vi "Main.vi"(11 "Module Admin":refnum<class "Delacor_lib_QMH_Module Admin.lvclass">) -> ()   [LabVIEW 2020, in "UI.lvlib"]
doc: "This template is based off of the Queued Message Handler design pattern and the Queued Message Handler project template that ships with LabVIEW.\n\nThe main difference is that the queue is private to this module and communication between modules is performed via Broadcast and Request events.\n\nRequest events are wrapped in public API methods and are handled in the Event Handling Loop (EHL) of this VI. Any module can register for Broadcast events sent by this module. The EHL generates messages based on user interface actions.\n\nThe Message Handling Loop (MHL) processes messages generated by the EHL, or by other messages. The messages are string values, so new messages can be added easily to the Message Cases case structure in the MHL. Each message cluster can also provide an optional value for Message Data, which is a variant that can be converted to whatever message-specific data is required.\n_____\nBased on Delacor QMH Project Template 5.0.0.82."
uses:
  UI.lvlib
  <vilib>/Delacor/Delacor QMH/Libraries/Module Admin_class/Delacor_lib_QMH_Module Admin.lvclass
  Module Data--cluster.ctl
  Stop Argument--cluster.ctl
  <vilib>/Delacor/Delacor QMH/Libraries/Message Queue_class/Delacor_lib_QMH_Message Queue.lvclass/Delacor_lib_QMH_Message Queue.ctl
  <vilib>/Delacor/Delacor QMH/Libraries/Module Admin_class/Delacor_lib_QMH_Module Admin.lvclass/Delacor_lib_QMH_Module Admin.ctl
  <vilib>/Delacor/Delacor QMH/Libraries/Message Queue_class/Delacor_lib_QMH_Enqueue Message (Single).vi
  <vilib>/Delacor/Delacor QMH/Libraries/Module Admin_class/Delacor_lib_QMH_Get External Launch.vi
  <vilib>/Utility/error.llb/Error Cluster From Error Code.vi
  <vilib>/ErrorRing/Error Ring.xnode
  <vilib>/Delacor/Delacor QMH/Libraries/Message Queue_class/Delacor_lib_QMH_Message Queue.lvclass
  Productos/Productos.lvlib
  Monedas/Monedas.lvlib
  Mensajes/Mensajes.lvlib
panel:
  out "error out":errorcluster
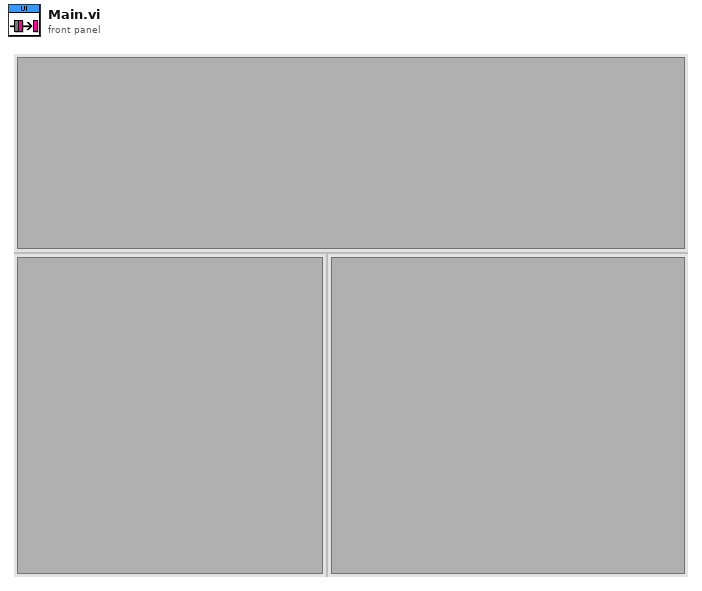
[diagram p1: front panel]
types:
  T1 = typedef "UI.lvlib/Request Events--cluster.ctl" = cluster{"Stop Module":refnum<user-event>, "Show Panel":refnum<user-event>, "Hide Panel":refnum<user-event>, "Get Module Execution Status":refnum<user-event>, "Show Diagram":refnum<user-event>}
  T2 = typedef "Mensajes.lvlib/Broadcast Events--cluster.ctl" = cluster{"Module Did Init":refnum<user-event>, "Status Updated":refnum<user-event>, "Error Reported":refnum<user-event>, "Module Did Stop":refnum<user-event>, "Update Module Execution Status":refnum<user-event>}
  T3 = typedef "Monedas.lvlib/Broadcast Events--cluster.ctl" = cluster{"Module Did Init":refnum<user-event>, "Status Updated":refnum<user-event>, "Error Reported":refnum<user-event>, "Module Did Stop":refnum<user-event>, "Update Module Execution Status":refnum<user-event>}
  T4 = typedef "Productos.lvlib/Broadcast Events--cluster.ctl" = cluster{"Module Did Init":refnum<user-event>, "Status Updated":refnum<user-event>, "Error Reported":refnum<user-event>, "Module Did Stop":refnum<user-event>, "Update Module Execution Status":refnum<user-event>}
  T5 = typedef "UI.lvlib/Module Data--cluster.ctl" = cluster{"Status":string}
  T6 = enum32{"invalid lock state", "Not Locked", "Locked (No Password)", "Password-protected"}
  T7 = typedef "UI.lvlib/Stop Argument--cluster.ctl" = cluster{"Origin":string, "Exit via Stop Module Req?":bool, "Wait for Module to stop?":bool}
  T8 = enum32{"Invalid", "Standard", "Closed", "Hidden", "Minimized", "Maximized"}
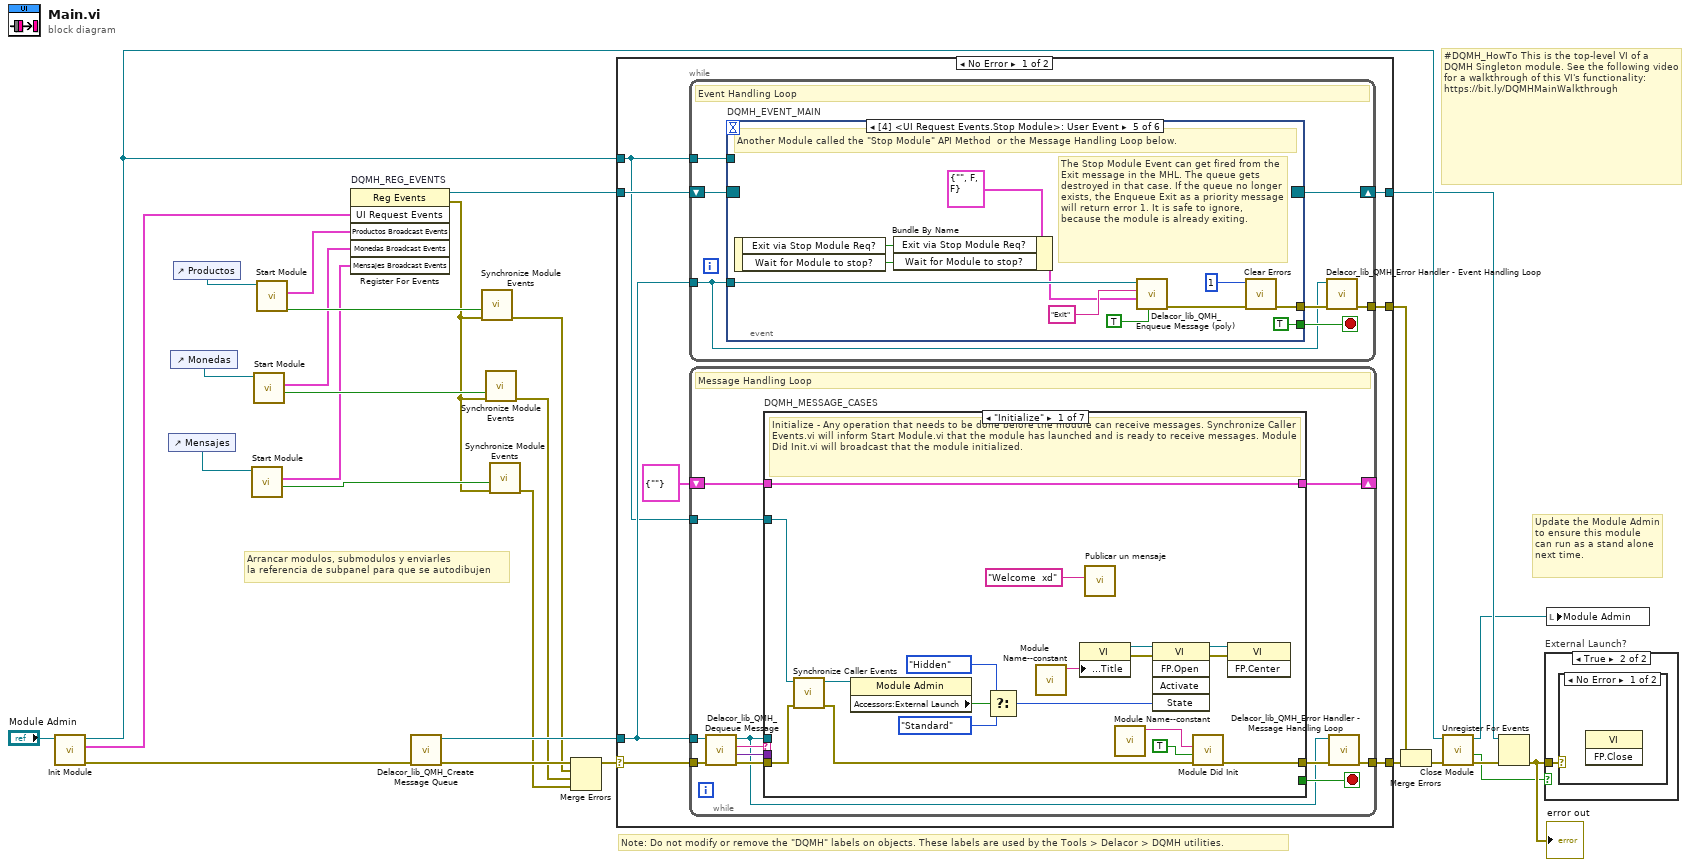
[diagram p0: block diagram]
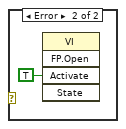
[diagram p3: hidden frame]
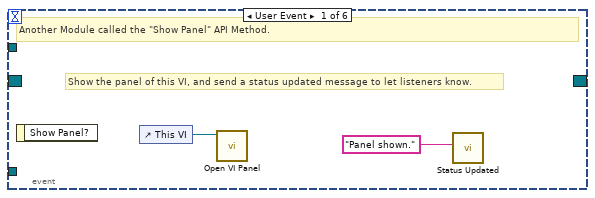
[diagram p4: hidden frame]
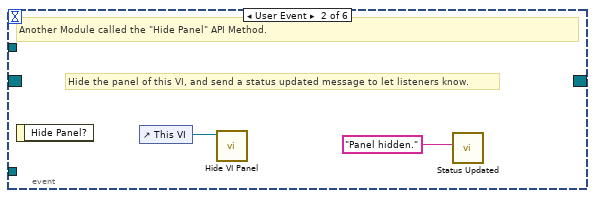
[diagram p5: hidden frame]
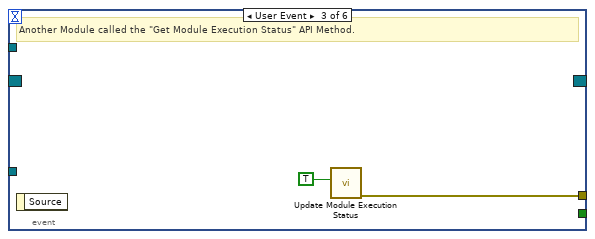
[diagram p6: hidden frame]
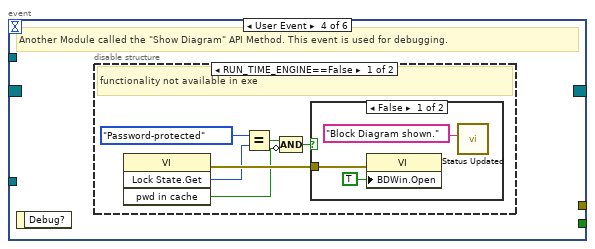
[diagram p7: hidden frame]
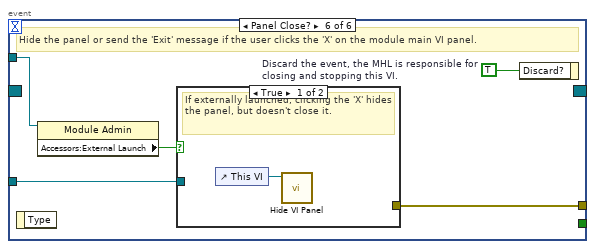
[diagram p10: hidden frame]
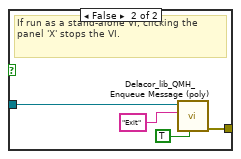
[diagram p11: hidden frame]
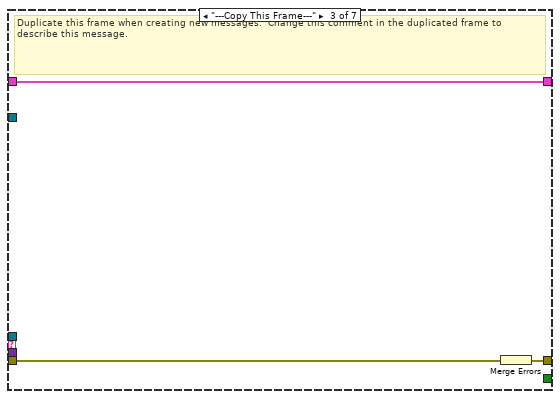
[diagram p13: hidden frame]
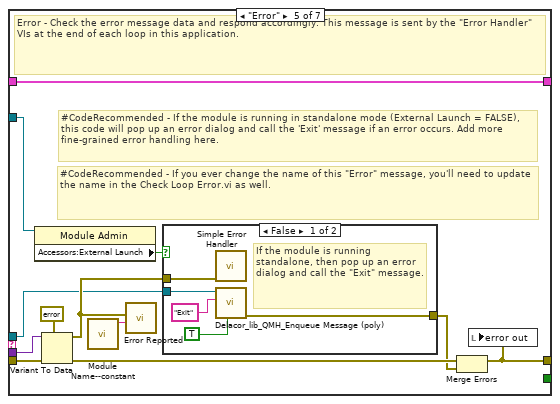
[diagram p15: hidden frame]
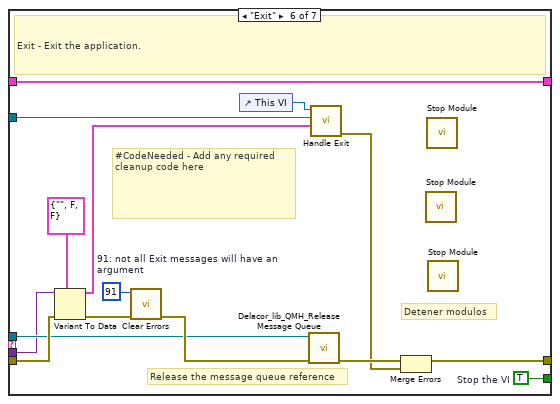
[diagram p17: hidden frame]
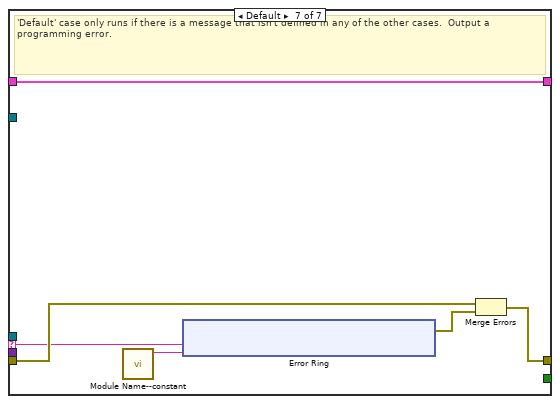
[diagram p18: hidden frame]
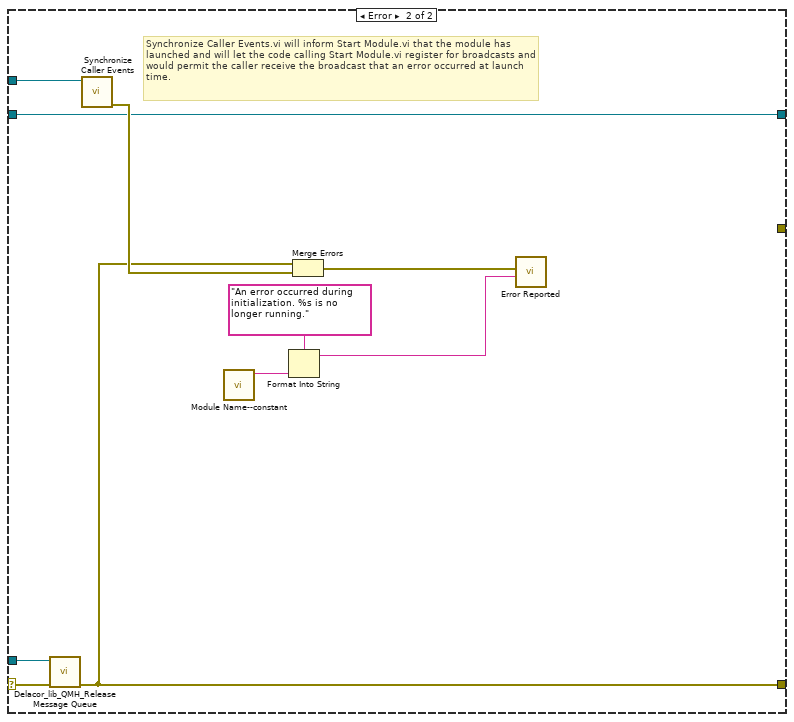
[diagram p19: hidden frame]
diagram:
  # "Arrancar modulos, submodulos y enviarles\nla referencia de subpanel para que se autodibujen"
  # "#DQMH_HowTo This is the top-level VI of a DQMH Singleton module. See the following video for a walkthrough of this VI's functionality: https://bit.ly/DQMHMainWalkthrough"
  # "Note: Do not modify or remove the \"DQMH\" labels on objects. These labels are used by the Tools > Delacor > DQMH utilities."
  # "Update the Module Admin to ensure this module can run as a stand alone next time."
  n1 = call "Init Module.vi"("Singleton Module Admin in"="Module Admin") -> ("error out"=w28:errorcluster, "UI Request Events"=w18:T1, "Singleton Module Admin out"=w21:refnum<class "Delacor_lib_QMH_Module Admin.lvclass">)  [unwired: 8 in]
  n2 = control-ref of="Mensajes"() -> (w7:refnum<vi>)
  n3 = control-ref of="Monedas"() -> (w10:refnum<vi>)
  n4 = control-ref of="Productos"() -> (w13:refnum<vi>)
  n5 = call "Start Module.vi"("Mensajes"=w7) -> ("Wait for Event Sync?"=w5:bool, "Mensajes Broadcast Events"=w6:T2)  [unwired: 7 in, 2 out]
  n6 = call "Start Module.vi"("Monedas"=w10) -> ("Wait for Event Sync?"=w8:bool, "Monedas Broadcast Events"=w9:T3)  [unwired: 7 in, 2 out]
  n7 = call "Start Module.vi"("Productos"=w13) -> ("Wait for Event Sync?"=w11:bool, "Productos Broadcast Events"=w12:T4)  [unwired: 7 in, 2 out]
  n8 = register-events "DQMH_REG_EVENTS"(w18, w12, w9, w6) -> (reference out=w19:refnum<event-registration>, error out=w4:errorcluster)  [unwired: 2 in]
  n9 = call <vilib>:"Delacor_lib_QMH_Create Message Queue.vi"("error in (no error)"=w28) -> ("error out"=w23:errorcluster, "Message Queue"=w17:refnum<class "Delacor_lib_QMH_Message Queue.lvclass">)  [unwired: 9 in]
  n10 = call "Synchronize Module Events.vi"("error in (no error)"=w4, "Wait for Event Sync?"=w11) -> ("error out"=w3:errorcluster)  [unwired: 9 in]
  n11 = call "Synchronize Module Events.vi"("error in (no error)"=w4, "Wait for Event Sync?"=w8) -> ("error out"=w2:errorcluster)  [unwired: 9 in]
  n12 = call "Synchronize Module Events.vi"("error in (no error)"=w4, "Wait for Event Sync?"=w5) -> ("error out"=w1:errorcluster)  [unwired: 9 in]
  n13 = Merge Errors(w23, w3, w2, w1) -> (w22:errorcluster)
  n14 = case shown="No Error" w22 {
    selector: w22 -> [w35 w166]
    tunnel: [w37 w165] -> w29
    tunnel: [w34 w171] -> w20
    tunnel: w19 -> [w32 w171]
    tunnel: w17 -> [w31 w164]
    tunnel: [w36 _] -> w26
    tunnel: w21 -> [w30 w167]
    frame No Error {
      n15 = while {
        tunnel: w31 -> [w38]
        shift-right: [w41] -> w34
        shift-left: w32 -> [w42]
        tunnel: [w43] -> w36
        tunnel: w30 -> [w39]
        stop <- w40 stop-if-true
        # "Event Handling Loop"
        n16 = event "DQMH_EVENT_MAIN" shown="[4] <UI Request Events.Stop Module>: User Event" {
          selector: w42 -> [_ _ _ _ _ _]
          dyn-events: [_ _ _ _ _ _] -> w41
          timeout: _ -> [_ _ _ _ _ _]
          tunnel: [_ _ _ _ TRUE ("Discard?") _] -> w40
          tunnel: w38 -> [_ _ _ _ w66 w73]
          tunnel: [_ _ w50 _ w69 w75] -> w44
          tunnel: w39 -> [_ _ _ _ _ w72]
          event User Event {
            # "Show the panel of this VI, and send a status updated message to let listeners know."
            # "Another Module called the \"Show Panel\" API Method."
            n17 = event-data() -> ()  [unwired: 1 in, 1 out]
            n18 = control-ref of="This VI"() -> (w46:refnum<vi>)
            n19 = call "Open VI Panel.vi"("VI"=w46) -> ()  [unwired: 10 in, 1 out]
            n20 = call "Status Updated.vi"("Status"="Panel shown." ("format string")) -> ()  [unwired: 10 in, 1 out]
          }
          event User Event {
            # "Hide the panel of this VI, and send a status updated message to let listeners know."
            # "Another Module called the \"Hide Panel\" API Method."
            n21 = event-data() -> ()  [unwired: 1 in, 1 out]
            n22 = control-ref of="This VI"() -> (w48:refnum<vi>)
            n23 = call "Hide VI Panel.vi"("VI"=w48) -> ()  [unwired: 10 in, 1 out]
            n24 = call "Status Updated.vi"("Status"="Panel hidden." ("format string")) -> ()  [unwired: 10 in, 1 out]
          }
          event User Event {
            # "Another Module called the \"Get Module Execution Status\" API Method."
            n25 = event-data() -> ()  [unwired: 1 in, 1 out]
            n26 = call "Update Module Execution Status.vi"("Running?"=TRUE) -> ("error out"=w50:errorcluster)  [unwired: 10 in]
          }
          event User Event {
            # "Another Module called the \"Show Diagram\" API Method. This event is used for debugging."
            n27 = event-data() -> ()  [unwired: 1 in, 1 out]
            n28 = disable-structure shown="RUN_TIME_ENGINE==False" {
              frame condition #0 (active) {
                # "functionality not available in exe"
                n29 = invoke class="VI" method="Lock State.Get"() -> (error out=w56:errorcluster, "Get Lock State"=w55:T6, "pwd in cache"=w52:bool)  [unwired: 4 in, 1 out]
                n30 = Equal?(x=T6."Password-protected", y=w55) -> (x = y?=w53:bool)
                n31 = Compound Arithmetic op=AND(w53, invert w52) -> (w51:bool)
                n32 = case shown="False" w51 {
                  tunnel: w56 -> [w59 _]
                  frame False {
                    n33 = property class="VI"(error in=w59, "BDWin.Open"=TRUE ("Block Diagram Window:Open")) -> ()  [unwired: 1 in, 2 out]
                    n34 = call "Status Updated.vi"("Status"="Block Diagram shown." ("format string")) -> ()  [unwired: 10 in, 1 out]
                  }
                  frame True {
                    # "Password-protected VI, and the password is not in the cache. Do not show the diagram."
                  }
                }
              }
              frame condition #1 {
              }
            }
          }
          event User Event {
            # "The Stop Module Event can get fired from the Exit message in the MHL. The queue gets destroyed in that case. If the queue no longer exists, the Enqueue Exit as a priority message will return error 1. It is safe to ignore, because the module is already exiting."
            # "Another Module called the \"Stop Module\" API Method  or the Message Handling Loop below."
            n35 = event-data() -> ("Exit via Stop Module Req?"=w62:bool, "Wait for Module to stop?"=w61:bool)  [unwired: 1 in]
            n36 = Bundle By Name(cluster=T7 {"Origin"="", "Exit via Stop Module Req?"=FALSE, "Wait for Module to stop?"=FALSE} ("Stop Argument"), "Exit via Stop Module Req?"=w62, "Wait for Module to stop?"=w61) -> (w60:T7)
            n37 = call-poly <vilib>:"Delacor_lib_QMH_Enqueue Message (poly).vi"("Priority Message? (F)"=TRUE, "Message Data"=w60, "Message"="Exit", "Message Queue in"=w66) -> ("error out"=w70:errorcluster)  [unwired: 6 in, 1 out]
            n38 = call <vilib>:"Clear Errors.vi"("error in (no error)"=w70, "specific error code to clear (0: all)"=1) -> ("error out"=w69:errorcluster)  [unwired: 4 in, 1 out]
          }
          event Panel Close? {
            w74 = TRUE  # Discard the event, the MHL is responsible for closing and stopping this VI.
            # "Hide the panel or send the 'Exit' message if the user clicks the 'X' on the module main VI panel."
            n39 = event-data() -> ()  [unwired: 1 in, 1 out]
            n40 = property class="Module Admin"(reference=w72) -> ("Accessors:External Launch"=w71:bool)  [unwired: 1 in, 2 out]
            n41 = case shown="True" w71 {
              tunnel: w73 -> [_ w79]
              tunnel: [_ w80] -> w75
              frame True {
                # "If externally launched, clicking the 'X' hides the panel, but doesn't close it."
                n42 = control-ref of="This VI"() -> (w76:refnum<vi>)
                n43 = call "Hide VI Panel.vi"("VI"=w76) -> ()  [unwired: 10 in, 1 out]
              }
              frame False {
                # "If run as a stand-alone VI, clicking the panel 'X' stops the VI."
                n44 = call-poly <vilib>:"Delacor_lib_QMH_Enqueue Message (poly).vi"("Priority Message? (F)"=TRUE, "Message"="Exit", "Message Queue in"=w79) -> ("error out"=w80:errorcluster)  [unwired: 7 in, 1 out]
              }
            }
            n45 = event-data("Discard?"=w74) -> ()  [unwired: 1 in, 1 out]
          }
        }
        n46 = call-dynamic "Delacor_lib_QMH_Error Handler - Event Handling Loop.vi"("error in (no error)"=w44, "Message Queue in"=w38) -> ("dup error in"=w43:errorcluster)  [unwired: 8 in, 1 out]
      }
      n47 = while {
        tunnel: w31 -> [w83]
        shift-right: [w87] -> _
        shift-left: T5 {"Status"=""} ("Data Cluster") -> [w88]
        tunnel: w35 -> [w91]
        tunnel: [w89] -> w37
        tunnel: w30 -> [w81]
        stop <- w86 stop-if-true
        # "Message Handling Loop"
        n48 = call-dynamic "Delacor_lib_QMH_Dequeue Message.vi"("error in (no error)"=w91, "Message Queue in"=w83) -> ("error out"=w90:errorcluster, "Message Data"=w84:variant, "Message"=w85:string, "Message Queue out"=w82:refnum<class "Delacor_lib_QMH_Message Queue.lvclass">)  [unwired: 6 in]
        n49 = case "DQMH_MESSAGE_CASES" shown="\"Initialize\"" w85 {
          selector: w85 -> [_ _ _ _ _ _ w151]
          tunnel: w82 -> [_ _ _ _ w121 w143 _]
          tunnel: w90 -> [w108 w112 w115 w117 w128 w149 w153]
          tunnel: [w106 w112 w114 w117 w124 w146 w154] -> w92
          tunnel: w88 -> [w97 w111 w113 w116 w123 w142 w152]
          tunnel: [w97 w111 w113 w116 w123 w142 w152] -> w87
          tunnel: [_ _ _ _ _ w141 _] -> w86
          tunnel: w84 -> [_ _ _ _ w122 w140 _]
          tunnel: w81 -> [w98 _ _ _ w120 w135 _]
          frame "Initialize" {
            # "Initialize - Any operation that needs to be done before the module can receive messages. Synchronize Caller Events.vi will inform Start Module.vi that the module has launched and is ready to receive messages. Module Did Init.vi will broadcast that the module initialized."
            n50 = call "Synchronize Caller Events.vi"("error in (no error)"=w108, "Singleton Module Admin in"=w98) -> ("error out"=w107:errorcluster, "Singleton Module Admin out"=w94:refnum<class "Delacor_lib_QMH_Module Admin.lvclass">)  [unwired: 8 in]
            n51 = property class="Module Admin"(reference=w94) -> ("Accessors:External Launch"=w102:bool)  [unwired: 1 in, 2 out]
            n52 = Select(t=T8."Hidden" ("State"), s=w102, f=T8."Standard" ("State")) -> (s? t:f=w99:T8)
            n53 = call "Module Name--constant.vi"() -> ("Module Name"=w105:string)  [unwired: 11 in]
            n54 = property class="VI"("Front Panel.Title"=w105) -> (reference out=w104:refnum<vi>, error out=w110:errorcluster)  [unwired: 2 in]
            n55 = call "Publicar un mensaje.vi"("Mensaje"="Welcome  xd") -> ()  [unwired: 10 in, 1 out]
            n56 = call "Module Name--constant.vi"() -> ("Module Name"=w95:string)  [unwired: 11 in]
            n57 = invoke class="VI" method="FP.Open"(reference=w104, error in=w110, "State"=w99) -> (reference out=w103:refnum<vi>, error out=w109:errorcluster)  [unwired: 2 in, 3 out]
            n58 = call "Module Did Init.vi"("error in (no error)"=w107, "Initialized?"=TRUE, "Origin"=w95) -> ("error out"=w106:errorcluster)  [unwired: 8 in]
            n59 = invoke class="VI" method="FP.Center"(reference=w103, error in=w109) -> ()  [unwired: 1 in, 3 out]
          }
          frame "--- Module Specific ---" {
            # "Separator -- The following cases handle messages specific to this Module."
          }
          frame "---Copy This Frame---" {
            # "Duplicate this frame when creating new messages.  Change this comment in the duplicated frame to describe this message."
            n60 = Merge Errors(w115) -> (w114:errorcluster)
          }
          frame "--- Exit and Error Handling---" {
            # "Separator - The following cases handle errors and exit messages."
          }
          frame "Error" {
            # "#CodeRecommended - If you ever change the name of this \"Error\" message, you'll need to update the name in the Check Loop Error.vi as well."
            # "#CodeRecommended - If the module is running in standalone mode (External Launch = FALSE), this code will pop up an error dialog and call the 'Exit' message if an error occurs. Add more fine-grained error handling here."
            # "Error - Check the error message data and respond accordingly. This message is sent by the \"Error Handler\" VIs at the end of each loop in this application."
            n61 = property class="Module Admin"(reference=w120) -> ("Accessors:External Launch"=w119:bool)  [unwired: 1 in, 2 out]
            n62 = Variant To Data(error in=w128, type=errorcluster {"status"=FALSE, "code"=0, "source"=""} ("error constant"), Variant=w122) -> (data=w129:errorcluster, error out=w126:errorcluster)
            n63 = call "Module Name--constant.vi"() -> ("Module Name"=w118:string)  [unwired: 11 in]
            n64 = call "Error Reported.vi"("Additional Information"=w118, "Error"=w129) -> ()  [unwired: 9 in, 1 out]
            n65 = case shown="False" w119 {
              tunnel: [w134 _] -> w125
              tunnel: w121 -> [w132 _]
              tunnel: w129 -> [w133 _]
              frame False {
                # "If the module is running standalone, then pop up an error dialog and call the \"Exit\" message."
                n66 = call <vilib>:"Simple Error Handler.vi"("error in (no error)"=w133) -> ()  [unwired: 4 in, 5 out]
                n67 = call-poly <vilib>:"Delacor_lib_QMH_Enqueue Message (poly).vi"("Priority Message? (F)"=TRUE, "Message"="Exit", "Message Queue in"=w132) -> ("error out"=w134:errorcluster)  [unwired: 7 in, 1 out]
              }
              frame True {
                # "If the module was launched externally, calling the Error Reported broadcast VI is the only action performed by the \"Error\" message. The module's caller can then process the error appropriately."
              }
            }
            n68 = Merge Errors(w126, w125) -> (w124:errorcluster)
            n69 = local write "error out"(w124) -> ()
          }
          frame "Exit" {
            w139 = 91  # 91: not all Exit messages will have an argument
            w141 = TRUE  # Stop the VI
            # "Detener modulos"
            # "Release the message queue reference"
            # "#CodeNeeded - Add any required cleanup code here"
            # "Exit - Exit the application."
            n70 = Variant To Data(error in=w149, type=T7 {"Origin"="", "Exit via Stop Module Req?"=FALSE, "Wait for Module to stop?"=FALSE} ("Stop Argument"), Variant=w140) -> (data=w137:T7, error out=w145:errorcluster)
            n71 = call <vilib>:"Clear Errors.vi"("error in (no error)"=w145, "specific error code to clear (0: all)"=w139) -> ("error out"=w148:errorcluster)  [unwired: 4 in, 1 out]
            n72 = control-ref of="This VI"() -> (w136:refnum<vi>)
            n73 = call-dynamic "Delacor_lib_QMH_Release Message Queue.vi"("error in (no error)"=w148, "Message Queue"=w143) -> ("error out"=w147:errorcluster)  [unwired: 9 in]
            n74 = call "Handle Exit.vi"("Stop Argument"=w137, "Admin in"=w135, "VI reference"=w136) -> ("error out"=w144:errorcluster)  [unwired: 7 in, 1 out]
            n75 = Merge Errors(w147, w144) -> (w146:errorcluster)
            n76 = call "Stop Module.vi"() -> ()  [unwired: 11 in, 1 out]
            n77 = call "Stop Module.vi"() -> ()  [unwired: 11 in, 1 out]
            n78 = call "Stop Module.vi"() -> ()  [unwired: 11 in, 1 out]
          }
          frame Default {
            # "'Default' case only runs if there is a message that isn't defined in any of the other cases.  Output a programming error."
            n79 = call "Module Name--constant.vi"() -> ("Module Name"=w150:string)  [unwired: 11 in]
            n80 = xnode "Error Ring"("parameter 0"=w151, "parameter 1"=w150) -> ("error out"=w155:errorcluster)
            n81 = Merge Errors(w153, w155) -> (w154:errorcluster)
          }
        }
        n82 = call-dynamic "Delacor_lib_QMH_Error Handler - Message Handling Loop.vi"("error in (no error)"=w92, "Message Queue in"=w82) -> ("dup error in"=w89:errorcluster)  [unwired: 8 in, 1 out]
      }
    }
    frame Error {
      # "Synchronize Caller Events.vi will inform Start Module.vi that the module has launched and will let the code calling Start Module.vi register for broadcasts and would permit the caller receive the broadcast that an error occurred at launch time."
      n83 = call-dynamic "Delacor_lib_QMH_Release Message Queue.vi"("error in (no error)"=w166, "Message Queue"=w164) -> ("error out"=w165:errorcluster)  [unwired: 9 in]
      n84 = call "Synchronize Caller Events.vi"("Singleton Module Admin in"=w167) -> ("error out"=w172:errorcluster)  [unwired: 9 in, 1 out]
      n85 = call "Module Name--constant.vi"() -> ("Module Name"=w170:string)  [unwired: 11 in]
      n86 = Format Into String(format string="An error occurred during initialization. %s is no longer running.", w170) -> (resulting string=w168:string)  [unwired: 2 in, 1 out]
      n87 = Merge Errors(w165, w172) -> (w173:errorcluster)
      n88 = call "Error Reported.vi"("Additional Information"=w168, "Error"=w173) -> ()  [unwired: 9 in, 1 out]
    }
  }
  n89 = Merge Errors(w26, w29) -> (w25:errorcluster)
  n90 = call "Close Module.vi"("error in (no error)"=w25, "Module Admin in"=w21) -> ("error out"=w27:errorcluster, "External Launch"=w14:bool, "Module Admin out"=w15:refnum<class "Delacor_lib_QMH_Module Admin.lvclass">)  [unwired: 7 in]
  n91 = Unregister For Events(event registration refnum=w20, error in=w27) -> (error out=w24:errorcluster)
  "error out" <- w24
  n92 = case "External Launch?" shown="True" w14 {
    tunnel: w24 -> [_ w174]
    frame False {
    }
    frame True {
      n93 = case shown="No Error" w174 {
        frame No Error {
          n94 = invoke class="VI" method="FP.Close"() -> ()  [unwired: 3 in, 3 out]
        }
        frame Error {
          n95 = invoke class="VI" method="FP.Open"("Activate"=TRUE ("Activate?")) -> ()  [unwired: 4 in, 5 out]
        }
      }
    }
  }
  n96 = local write "Module Admin"(w15) -> ()
